vi "Get Command Infos.vi"(8 "error in (no error)":errorcluster, 11 "Input Device in":refnum<class "Input Device.lvclass">) -> (0 "error out":errorcluster, 3 "Input Device out":refnum<class "Input Device.lvclass">, 4 "Direction info out":string, 6 "Boost info out":string)   [LabVIEW 2021, in "Input Device.lvclass"]
doc: "MIT Licence\nCopyright (c) 2024 David Grollier"
uses:
  Input Device.lvclass
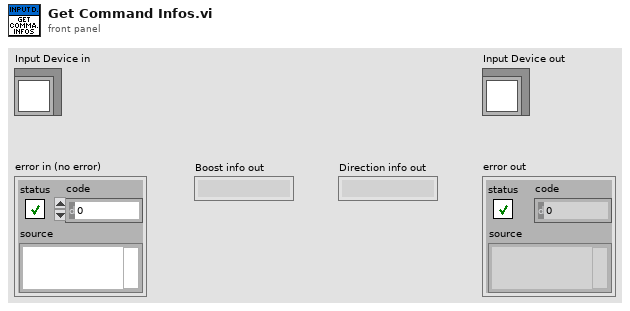
[diagram p1: front panel]
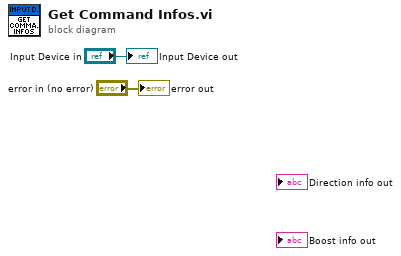
[diagram p0: block diagram]
diagram:
  "error out" <- "error in (no error)"
  "Input Device out" <- "Input Device in"
